vi "REPORT_CBATCH_listbox_set_values_and_recolor.vi"(7 "column_names":string[](array[string]), 8 "error_in":errorcluster, 10 "order":enum32{"old_to_new", "new_to_old"}(ring), 11 "REPORT_all_info_in":T1) -> (0 "error_out":errorcluster, 3 "REPORT_all_info_out":T1)   [LabVIEW 2019]
uses:
  FGV/REPORTS_records_display/REPORTS_all_info.ctl
  GEAR/typedef/REPORT_GEAR_all_info.ctl
  GEAR/typedef/REPORT_GEAR_header_data_display.ctl
  GEAR/typedef/REPORT_GEAR_statuses.ctl
  DATES/typedef/REPORT_DATES_all_info.ctl
  DATES/typedef/REPORT_DATES_statuses.ctl
  PRODUCTION_BATCH/typedef/REPORT_PBATCH_all_info.ctl
  OPERATION/typedef/REPORT_OPRTN_all_info.ctl
  CONFIG_HISTORY/typedef/REPORT_CFG_all_info.ctl
  CONFIG_HISTORY/typedef/REPORT_CFG_types.ctl
  AUDIT/typedef/REPORT_AUDIT_all_info.ctl
  OK_NOK_COUNT/typedef/REPORT_OKNOK_all_info.ctl
  REWORKS/typedef/REPORT_REWORKS_all_info.ctl
  PACE/typedef/REPORT_PACE_all_info.ctl
  typedef/REPORT_CBATCH_all_info.ctl
  GEAR_COMPONENTS/typedef/REPORT_CMPNT_all_info.ctl
  FGV/REPORTS_records_display/REPORTS_references.ctl
  <vilib>/Utility/miscctls.llb/LVRowAndColumnTypeDef.ctl
  <vilib>/Utility/miscctls.llb/LVRowAndColumnUnsignedTypeDef.ctl
  <userlib>/_OpenG.lib/array/array.llb/Reverse 2D Array (String)__ogtk.vi
panel:
  # "GEAR INFO SUMMARY"
  # "GEAR INFO SUMMARY"
  # "GEAR INFO SUMMARY"
  # "GEAR INFO SUMMARY"
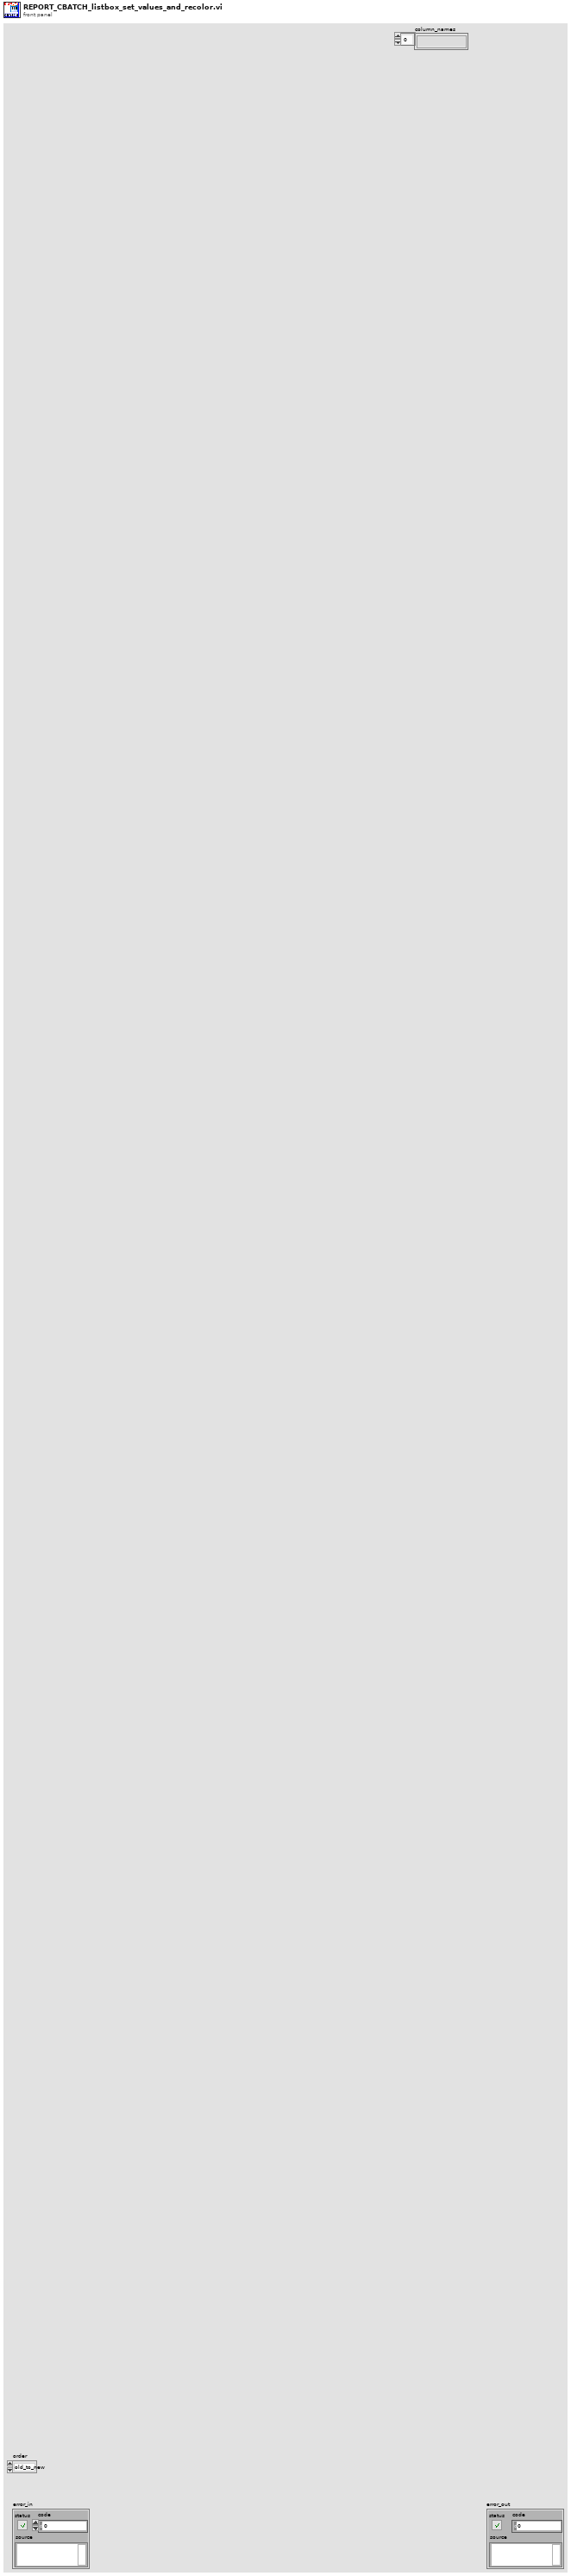
[diagram p1: front panel]
types:
  T1 = typedef "REPORTS_all_info.ctl" = cluster{"REPORT_GEAR_all_info":T2, "REPORT_DATES_all_info":T5, "REPORT_PBATCH_all_info":T7, "REPORT_OPRTN_all_info":T8, "REPORT_CFG_all_info":T9, "REPORT_AUDIT_all_info":T11, "REPORT_OKNOK_all_info":T12, "REPORT_REWORKS_all_info":T13, "REPORT_PACE_all_info":T14, "REPORT_CBATCH_all_info":T15, "REPORT_CMPNT_all_info":T16, "REPORTS_references":T17}
  T2 = typedef "REPORT_GEAR_all_info.ctl" = cluster{"serial":string, "filter_OP":string, "REPORT_GEAR_header":T3, "operations":string[][], "operation_statuses":T4[], "results":string[][], "result_statuses":T4[], "batches":string[][], "batch_statuses":T4[], "column_headers":string[], "displayed_rows":string[][], "displayed_statuses":T4[], "column_widths":i16[]}
  T3 = typedef "REPORT_GEAR_header_data_display.ctl" = cluster{"ID":string, "creation_time":string, "last_station":string, "last_status":string, "pinion_serial":string, "batch_code":string}
  T4 = typedef "REPORT_GEAR_statuses.ctl" = enum16{"OP_OK_hide", "OP_OK_show", "OP_NOK_hide", "OP_NOK_show", "OP_interrupted_hide", "OP_interrupted_show", "OP_in_operation_hide", "OP_in_operation_show", "OP_unexpected_hide", "OP_unexpected_show", "RE_REAL_OK", "RE_REAL_NOK", "RE_STRING", "RE_sub_header", "RE_no_data", "RE_unexpected", "BA_sub_header", "BA_data", "BA_no_data"}
  T5 = typedef "REPORT_DATES_all_info.ctl" = cluster{"date_start":string, "date_end":string, "time_start":string, "time_end":string, "filter_last_OP":string, "filter_last_status":string, "gears":string[][], "gears_statuses":T6[], "column_headers":string[], "displayed_rows":string[][], "displayed_statuses":T6[], "column_widths":i16[], "active_page":i32}
  T6 = typedef "REPORT_DATES_statuses.ctl" = enum16{"GEAR_OK", "GEAR_NOK", "GEAR_interrupted", "GEAR_in_operation", "GEAR_unexpected"}
  T7 = typedef "REPORT_PBATCH_all_info.ctl" = cluster{"batch_no":string, "filter_last_OP":string, "filter_last_status":string, "gears":string[][], "gears_statuses":T6[], "column_headers":string[], "displayed_rows":string[][], "displayed_statuses":T6[], "column_widths":i16[], "active_page":i32}
  T8 = typedef "REPORT_OPRTN_all_info.ctl" = cluster{"OP":string, "date_start":string, "date_end":string, "time_start":string, "time_end":string, "filter_last_status":string, "no_of_static_columns":i32, "operations":string[][], "operations_statuses":T6[], "column_headers":string[], "archivisation_description":string[][], "displayed_rows":string[][], "displayed_statuses":T6[], "column_widths":i16[], "hidden_columns":i32[], "active_page":i32}
  T9 = typedef "REPORT_CFG_all_info.ctl" = cluster{"type":T10, "date_start":string, "date_end":string, "time_start":string, "time_end":string, "filter_OP":string, "records":string[][], "column_headers":string[], "displayed_rows":string[][], "column_widths":i16[], "active_page":i32}
  T10 = typedef "REPORT_CFG_types.ctl" = enum16{"REFERENCE", "ARCHIVISATION", "USERS"}
  T11 = typedef "REPORT_AUDIT_all_info.ctl" = cluster{"date_start":string, "date_end":string, "time_start":string, "time_end":string, "filter_OP":string, "filter_status":string, "records":string[][], "record_statuses":T6[], "column_headers":string[], "displayed_rows":string[][], "displayed_statuses":T6[], "column_widths":i16[], "active_page":i32}
  T12 = typedef "REPORT_OKNOK_all_info.ctl" = cluster{"date_start":string, "date_end":string, "time_start":string, "time_end":string, "records":string[][], "column_headers":string[], "column_widths":i16[]}
  T13 = typedef "REPORT_REWORKS_all_info.ctl" = cluster{"date_start":string, "date_end":string, "time_start":string, "time_end":string, "from_OP":string, "to_OP":string, "records":string[][], "record_statuses":T6[], "column_headers":string[], "displayed_rows":string[][], "displayed_statuses":T6[], "column_widths":i16[], "active_page":i32}
  T14 = typedef "REPORT_PACE_all_info.ctl" = cluster{"date_start":string, "date_end":string, "time_start":string, "time_end":string, "low_limit":u16, "high_limit":u16, "records":string[][], "column_headers":string[], "column_widths":i16[]}
  T15 = typedef "REPORT_CBATCH_all_info.ctl" = cluster{"batch_code":string, "records":string[][], "record_statuses":T6[], "column_headers":string[], "displayed_rows":string[][], "displayed_statuses":T6[], "column_widths":i16[], "active_page":i32}
  T16 = typedef "REPORT_CMPNT_all_info.ctl" = cluster{"gear_serial":string, "records":string[][], "column_headers":string[], "displayed_rows":string[][], "column_widths":i16[], "active_page":i32}
  T17 = typedef "REPORTS_references.ctl" = cluster{"front_panel_reference":refnum<vi>, "SQL_listbox_reference":refnum<vi>, "REPORT_page_first":refnum<vi>, "REPORT_page_previous":refnum<vi>, "REPORT_page_next":refnum<vi>, "REPORT_page_last":refnum<vi>, "REPORT_page_counter":refnum<vi>, "REPORT_GEAR_serial":refnum<vi>, "REPORT_GEAR_serial_display":refnum<vi>, "REPORT_GEAR_station":refnum<vi>, "REPORT_GEAR_header_data_display":refnum<vi>, "REPORT_DATES_start":refnum<vi>, "REPORT_DATES_end":refnum<vi>, "REPORT_DATES_time_start":refnum<vi>, "REPORT_DATES_time_end":refnum<vi>, "REPORT_DATES_order_selection":refnum<vi>, "REPORT_DATES_last_OP":refnum<vi>, "REPORT_DATES_last_status":refnum<vi>, "REPORT_PBATCH_batch_no":refnum<vi>, "REPORT_PBATCH_order_selection":refnum<vi>, "REPORT_PBATCH_last_op":refnum<vi>, "REPORT_PBATCH_last_status":refnum<vi>, "REPORT_OPRTN_operation":refnum<vi>, "REPORT_OPRTN_start":refnum<vi>, "REPORT_OPRTN_end":refnum<vi>, "REPORT_OPRTN_time_start":refnum<vi>, "REPORT_OPRTN_time_end":refnum<vi>, "REPORT_OPRTN_order_selection":refnum<vi>, "REPORT_OPRTN_last_status":refnum<vi>, "REPORT_CFG_type":refnum<vi>, "REPORT_CFG_start":refnum<vi>, "REPORT_CFG_end":refnum<vi>, "REPORT_CFG_time_start":refnum<vi>, "REPORT_CFG_time_end":refnum<vi>, "REPORT_CFG_order_selection":refnum<vi>, "REPORT_CFG_op_filter":refnum<vi>, "REPORT_AUDIT_start":refnum<vi>, "REPORT_AUDIT_end":refnum<vi>, "REPORT_AUDIT_time_start":refnum<vi>, "REPORT_AUDIT_time_end":refnum<vi>, "REPORT_AUDIT_order_selection":refnum<vi>, "REPORT_AUDIT_op_filter":refnum<vi>, "REPORT_AUDIT_status_filter":refnum<vi>, "REPORT_OKNOK_start":refnum<vi>, "REPORT_OKNOK_end":refnum<vi>, "REPORT_OKNOK_time_start":refnum<vi>, "REPORT_OKNOK_time_end":refnum<vi>, "REPORT_REWORKS_start":refnum<vi>, "REPORT_REWORKS_end":refnum<vi>, "REPORT_REWORKS_time_start":refnum<vi>, "REPORT_REWORKS_time_end":refnum<vi>, "REPORT_REWORKS_from_OP":refnum<vi>, "REPORT_REWORKS_to_OP":refnum<vi>, "REPORT_REWORKS_order_selection":refnum<vi>, "REPORT_PACE_start":refnum<vi>, "REPORT_PACE_end":refnum<vi>, "REPORT_PACE_time_start":refnum<vi>, "REPORT_PACE_time_end":refnum<vi>, "REPORT_PACE_low_limit":refnum<vi>, "REPORT_PACE_high_limit":refnum<vi>, "REPORT_CBATCH_batch_code":refnum<vi>, "REPORT_CBATCH_order_selection":refnum<vi>, "REPORT_CMPNT_gear_serial":refnum<vi>}
  T18 = typedef "LVRowAndColumnUnsignedTypeDef.ctl" = cluster{"Row":u32, "Column":u32}
  T19 = typedef "LVRowAndColumnTypeDef.ctl" = cluster{"Row":i32, "Column":i32}
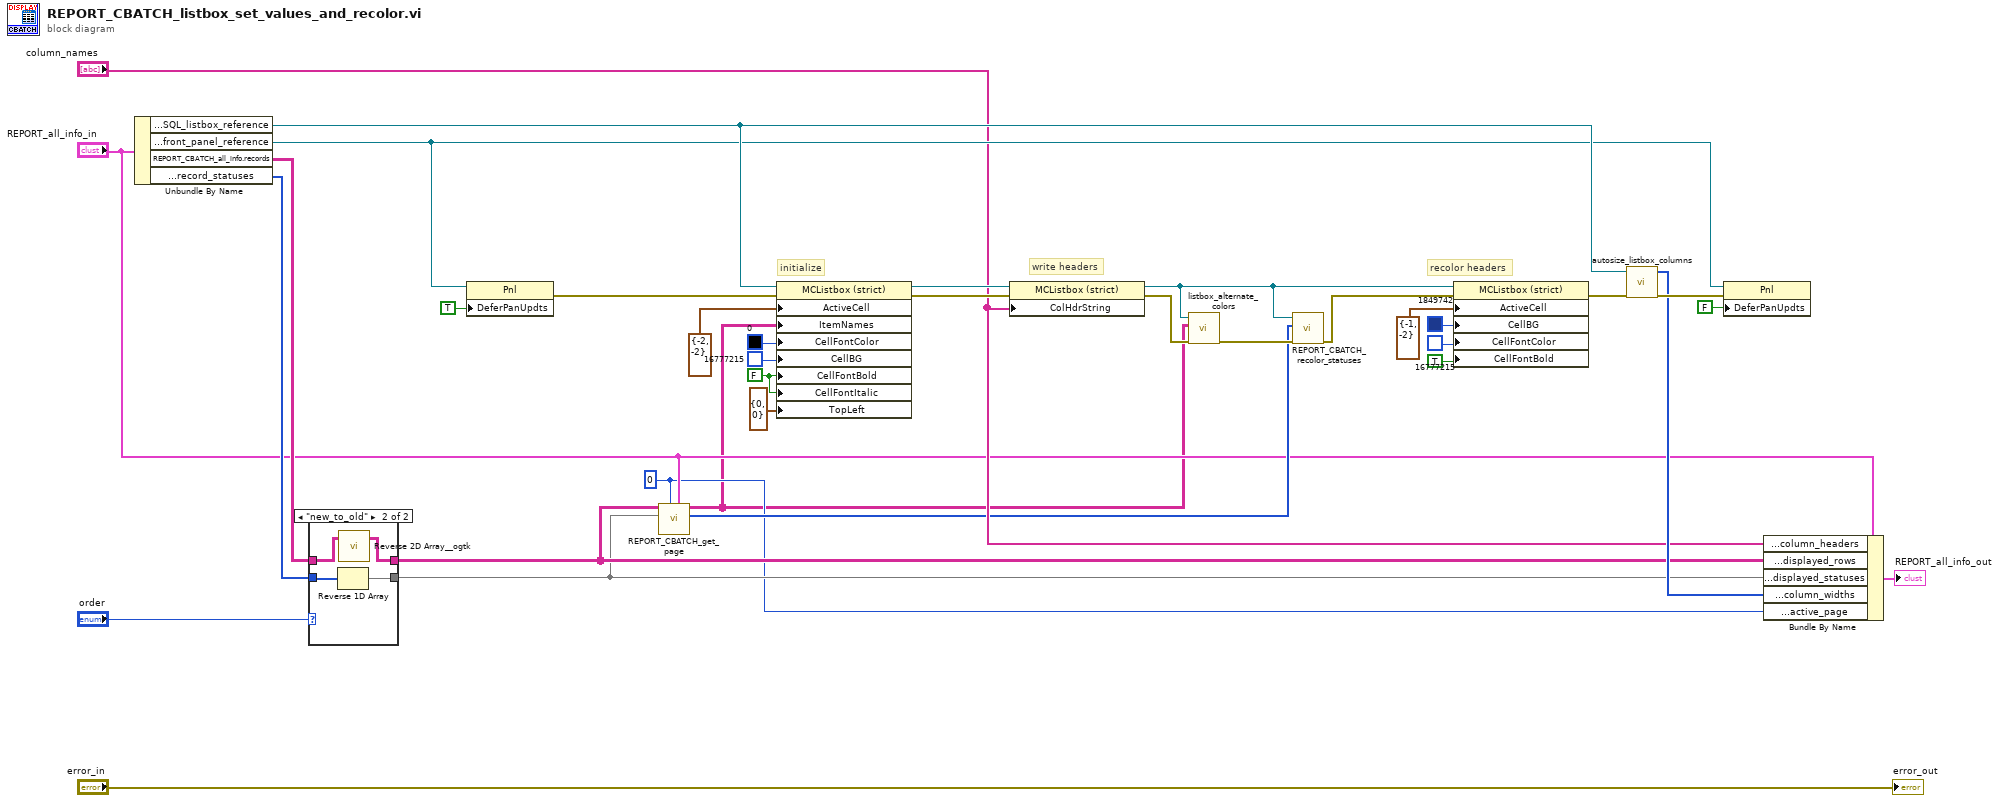
[diagram p0: block diagram]
diagram:
  w3 = 0
  w25 = FALSE ("Active Cell:Cell Font:Bold")
  # "recolor headers"
  # "initialize"
  # "write headers"
  n1 = Unbundle By Name("REPORT_all_info_in") -> ("REPORTS_references.SQL_listbox_reference"=w28:refnum<vi>, "REPORTS_references.front_panel_reference"=w27:refnum<vi>, "REPORT_CBATCH_all_info.records"=w9:string[][], "REPORT_CBATCH_all_info.record_statuses"=w8:T6[])
  n2 = case shown="\"new_to_old\"" "order" {
    tunnel: w9 -> [w37 w39]
    tunnel: [w37 w38] -> w7
    tunnel: w8 -> [w36 w41]
    tunnel: [w36 w40] -> w6
    frame "old_to_new" {
    }
    frame "new_to_old" {
      n3 = Reverse 1D Array(array=w41) -> (reversed array=w40:T6[])
      n4 = call-poly <userlib>:"Reverse 2D Array__ogtk.vi"("Array"=w39) -> ("Reversed Array"=w38:string[][])  [unwired: 2 in]
    }
  }
  n5 = property on="Property Node" class="Pnl"(reference=w27, "DeferPanUpdts"=TRUE ("Defer Panel Updates")) -> (error out=w1:errorcluster)  [unwired: 1 in, 1 out]
  n6 = call "REPORT_CBATCH_get_page.vi"("REPORT_all_info_in"="REPORT_all_info_in", "page_no"=w3, "gears_statuses"=w6, "gears"=w7) -> ("page_statuses"=w5:T6[], "page"=w2:string[][])  [unwired: 6 in]
  n7 = property on="Property Node" class="MCListbox (strict)"(reference=w28, error in=w1, "ActiveCell"=T19 {"Row"=-2, "Column"=-2} ("Active Cell:Active Cell"), "ItemNames"=w2, "CellFontColor"=u32 0, "CellBG"=u32 16777215, "CellFontBold"=w25, "CellFontItalic"=w25, "TopLeft"=T18 {"Row"=0, "Column"=0} ("Top Left Visible Cell")) -> (reference out=w31:refnum<vi>, error out=w29:errorcluster)
  n8 = property on="Property Node" class="MCListbox (strict)"(reference=w31, error in=w29, "ColHdrString"="column_names") -> (reference out=w18:refnum<vi>, error out=w16:errorcluster)
  n9 = call "listbox_alternate_colors.vi"("error_in"=w16, "item_names"=w2, "listbox_ref"=w18) -> ("error_out"=w17:errorcluster)  [unwired: 8 in]
  n10 = call "REPORT_CBATCH_recolor_statuses.vi"("error_in"=w17, "record_statuses"=w5, "listbox_ref"=w18) -> ("error_out"=w15:errorcluster)  [unwired: 8 in]
  n11 = property on="Property Node" class="MCListbox (strict)"(reference=w18, error in=w15, "ActiveCell"=T19 {"Row"=-1, "Column"=-2} ("Active Cell:Active Cell"), "CellBG"=u32 1849742, "CellFontColor"=u32 16777215, "CellFontBold"=TRUE ("Active Cell:Cell Font:Bold")) -> (error out=w33:errorcluster)  [unwired: 1 out]
  n12 = call "autosize_listbox_columns.vi"("error in (no error)"=w33, "Table Ref"=w28) -> ("error out"=w32:errorcluster, "column_widths"=w13:i16[])  [unwired: 4 in]
  n13 = property on="Property Node" class="Pnl"(reference=w27, error in=w32, "DeferPanUpdts"=FALSE ("Defer Panel Updates")) -> ()  [unwired: 2 out]
  n14 = Bundle By Name(cluster="REPORT_all_info_in", "REPORT_CBATCH_all_info.column_headers"="column_names", "REPORT_CBATCH_all_info.displayed_rows"=w7, "REPORT_CBATCH_all_info.displayed_statuses"=w6, "REPORT_CBATCH_all_info.column_widths"=w13, "REPORT_CBATCH_all_info.active_page"=w3) -> (→"REPORT_all_info_out":T1)
  "error_out" <- "error_in"
